vi "Climb (Piston) Controller.vi"(8 "error in":errorcluster) -> ()   [LabVIEW 2020]
doc: "This VI executes continuously carrying out the current operation and responding to updates or new operations. It will often contain the timing or control code that is difficult to place directly in TeleOp. This VI generally opens all sensors and motors and isolates the rest of the robot code from knowing how the operations are carried out."
uses:
  <vilib>/Rock Robotics/WPI/Framework/Completion Status.ctl
  Climb (Piston) Setpoints.ctl
  Climb (Piston) Operations.ctl
  <vilib>/Rock Robotics/WPI/Solenoid/WPI_SolenoidChannel.ctl
  <vilib>/Rock Robotics/WPI/Solenoid/WPI_SolenoidValue.ctl
  <vilib>/Rock Robotics/WPI/Solenoid/WPI_SolenoidOpenSingle.vi
  <vilib>/Rock Robotics/WPI/Solenoid/WPI_SolenoidSetEnum.vi
  <vilib>/Rock Robotics/Network Tables/NT Write Boolean.vi
panel:
  in  "Interactive Values":T1
  out "Current\nCmd":string
  in  "Buttons":cluster{"Execute Cmd":bool, "Abort Cmd":bool}
  out "Command Timing":cluster{"Start Time (ms)":u32, "Iterations":i32}
  out "Status":T3
  # "Tip: It may be helpful to observe inputs and sensor values.\nYou may also want to display tuning or debugging controls."
  # "Interactive Command: You may fill in the settings for a command\nand schedule it with the Execute button. You can observe and abort\nany command while fine tuning the code for the controller."
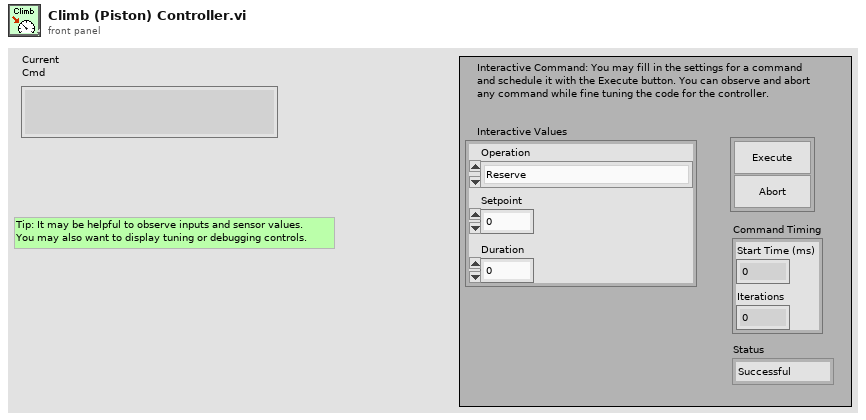
[diagram p1: front panel]
types:
  T1 = typedef "Climb (Piston) Setpoints.ctl" = cluster{"Operation":T2, "Setpoint":dbl, "Duration":dbl}
  T2 = typedef "Climb (Piston) Operations.ctl" = enum16{"Reserve", "Read Current", "Immediate", "Piston Up", "Piston Down"}
  T3 = typedef "Completion Status.ctl" = enum16{"Successful", "Aborted", "Incomplete"}
  T4 = typedef "WPI_SolenoidChannel.ctl" = enum8{"Solenoid 0", "Solenoid 1", "Solenoid 2", "Solenoid 3", "Solenoid 4", "Solenoid 5", "Solenoid 6", "Solenoid 7", "Solenoid 8", "Solenoid 9", "Solenoid 10", "Solenoid 11", "Solenoid 12", "Solenoid 13", "Solenoid 14", "Solenoid 15", "Invalid"}
  T5 = typedef "WPI_CompressorDevRef.ctl" = cluster{"DevStatus":errorcluster, "Pneumatics Control Module":u8}
  T6 = typedef "WPI_SolenoidDevRef.ctl" = cluster{"DevStatus":errorcluster, "Pneumatics Control Module":u8, "Forward Solenoid Channel":T4, "Reverse Solenoid Channel":T4}
  T7 = typedef "Command Status Info.ctl" = cluster{"Name":string, "Status":T3, "notifier out":T8}
  T8 = typedef "Completion Notifier.ctl" = refnum<notifier>
  T9 = cluster{"Current Command":T1, "Command Timing":cluster{"Start Time (ms)":u32, "Iterations":i32}, "Command Arguments":cluster{"Command Info":T7, "Description":string, "Default Command":T1, "queue out":refnum<queue>, "Subsystem Name":string}}
  T10 = typedef "WPI_SolenoidValue.ctl" = enum16{"Off", "On", "Forward", "Reverse"}
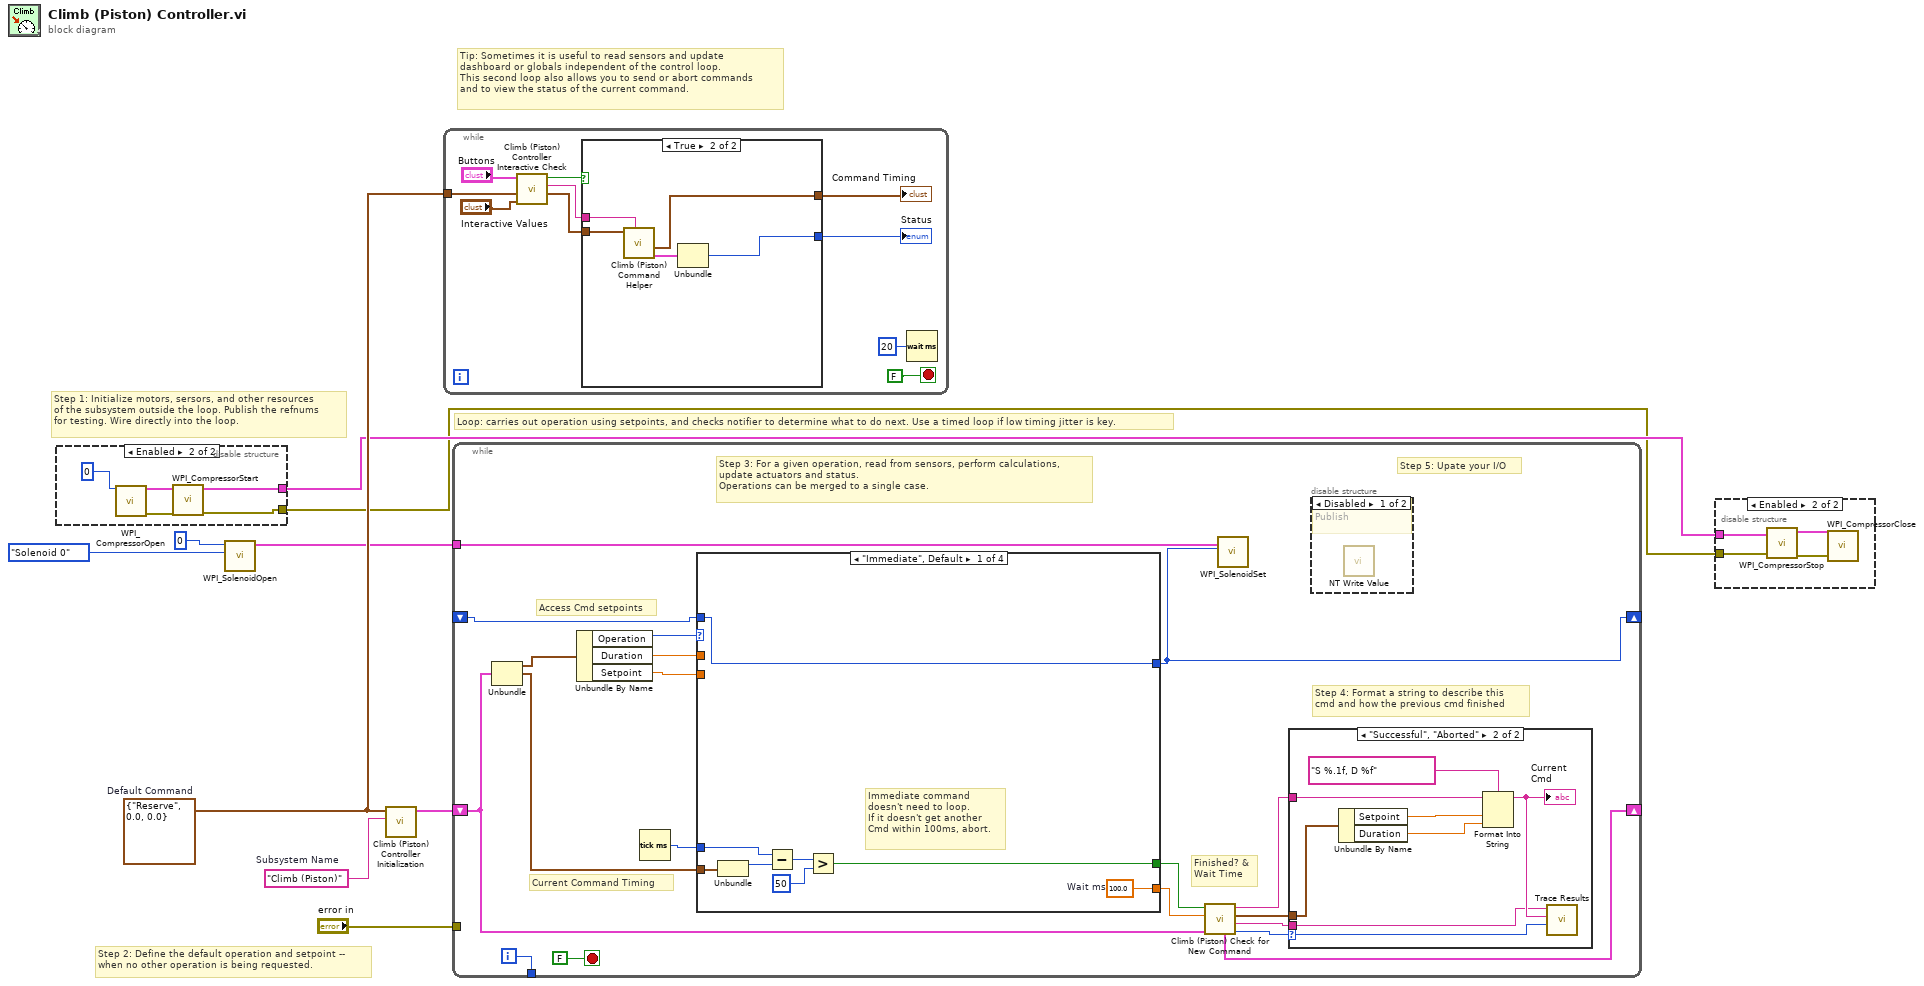
[diagram p0: block diagram]
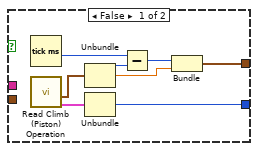
[diagram p4: hidden frame]
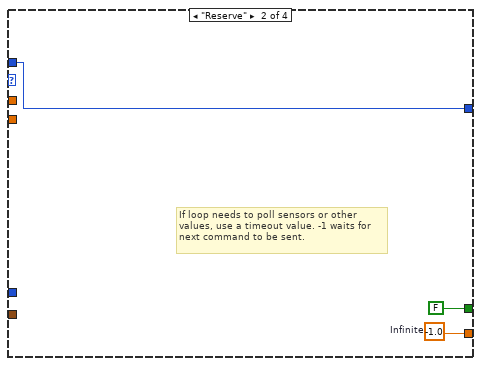
[diagram p7: hidden frame]
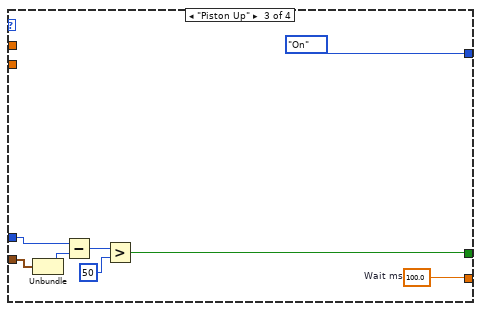
[diagram p8: hidden frame]
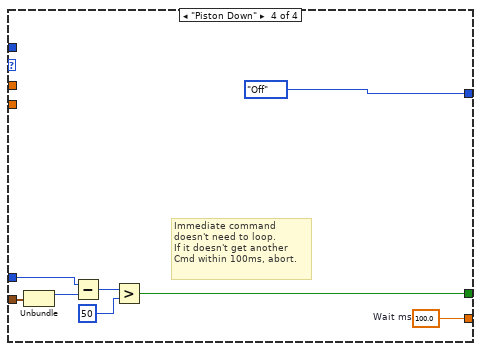
[diagram p9: hidden frame]
diagram:
  w6 = T1 {"Operation"=enum."Reserve", "Setpoint"=0.0, "Duration"=0.0}  # Default Command
  w7 = "Climb (Piston)"  # Subsystem Name
  # "Tip: Sometimes it is useful to read sensors and update\ndashboard or globals independent of the control loop.\nThis second loop also allows you to send or abort commands\nand to view the status of the current command."
  # "Step 2: Define the default operation and setpoint --\nwhen no other operation is being requested."
  # "Step 1: Initialize motors, sersors, and other resources\nof the subsystem outside the loop. Publish the refnums\nfor testing. Wire directly into the loop."
  # "Loop: carries out operation using setpoints, and checks notifier to determine what to do next. Use a timed loop if low timing jitter is key."
  n1 = disable-structure shown="Enabled" {
    disable-tunnel: [_ w12] -> w2
    disable-tunnel: [_ w11] -> w1
    frame Disabled {
    }
    frame Enabled {
      n2 = call <vilib>:"WPI_CompressorOpen.vi"("Pneumatics device (def)"=u8 0) -> ("CompressorDevRef"=w14:T5, "error out"=w13:errorcluster)  [unwired: 13 in]
      n3 = call <vilib>:"WPI_CompressorStart.vi"("error in (no error)"=w13, "CompressorDevRef"=w14) -> ("error out"=w11:errorcluster, "CompressorDevRef"=w12:T5)  [unwired: 8 in]
    }
  }
  n4 = call-poly <vilib>:"WPI_SolenoidOpen.vi"("Solenoid Channel"=WPI_SolenoidChannel."Solenoid 0", "Pneumatics Device (def)"=u8 0 ("Pneumatics Control Module (0)")) -> ("SolenoidDevRef"=w3:T6)  [unwired: 8 in, 1 out]
  n5 = call "Climb (Piston) Controller Initialization.vi"("Subsystem Name"=w7, "Default Command"=w6) -> ("Current Command"=w8:T9)  [unwired: 9 in]
  n6 = while {
    tunnel: w6 -> [w21]
    stop <- FALSE stop-if-true
    n7 = call "Climb (Piston) Controller Interactive Check.vi"("Interactive Command in"="Interactive Values", "Default Command"=w21, "Buttons"="Buttons") -> ("Interactive Command out"=w18:T1, "Trace String"=w19:string, "Schedule"=w20:bool)  [unwired: 6 in]
    n8 = case shown="True" w20 {
      tunnel: [w32 w37] -> w17
      tunnel: w18 -> [_ w35]
      tunnel: [w28 w33] -> w16
      tunnel: w19 -> [_ w36]
      frame False {
        n9 = Tick Count (ms)() -> (millisecond timer value=w27:u32)
        n10 = call "Read Climb (Piston) Operation.vi"() -> ("Command Info"=w25:T7, "SubSystem Data"=w26:T1)  [unwired: 9 in, 1 out]
        n11 = Unbundle(w26) -> ("Operation"=w31:T2, "Setpoint"=w29:dbl)  [unwired: 1 out]
        n12 = Unbundle(w25) -> ("Status"=w32:T3)  [unwired: 2 out]
        n13 = Subtract(x=w27, y=w31) -> (x-y=w30:u32)
        n14 = Bundle(w30, "Setpoint"=w29) -> (w28:cluster{u32, "Setpoint":dbl})  [unwired: 1 in]
      }
      frame True {
        n15 = call "Climb (Piston) Command Helper.vi"("Description"=w36, "SubSystem Data"=w35) -> ("Command Info Out"=w34:T7, "Command Timing"=w33:cluster{"Start Time (ms)":u32, "Iterations":i32})  [unwired: 7 in, 1 out]
        n16 = Unbundle(w34) -> ("Status"=w37:T3)  [unwired: 2 out]
      }
    }
    "Status" <- w17
    "Command Timing" <- w16
    n17 = Wait (ms)(milliseconds to wait=u32 20) -> ()  [unwired: 1 out]
  }
  n18 = while {
    shift-right: [w48] -> _
    shift-left: w8 -> [w41]
    tunnel: [w55] -> _
    tunnel: "error in" -> [_]
    tunnel: w3 -> [w40]
    shift-right: [w39] -> _
    shift-left: _ -> [w38]
    i -> [w55]
    stop <- FALSE stop-if-true
    # "Step 5: Upate your I/O"
    # "Step 4: Format a string to describe this\ncmd and how the previous cmd finished"
    # "Current Command Timing"
    # "Access Cmd setpoints"
    # "Finished? &\nWait Time"
    # "Step 3: For a given operation, read from sensors, perform calculations,\nupdate actuators and status.\nOperations can be merged to a single case."
    n19 = Unbundle(w41) -> ("Current Command"=w54:T1, "Command Timing"=w50:cluster{"Start Time (ms)":u32, "Iterations":i32})  [unwired: 1 out]
    n20 = Unbundle By Name(w54) -> ("Operation"=w53:T2, "Duration"=w52:dbl, "Setpoint"=w49:dbl)
    n21 = Tick Count (ms)() -> (millisecond timer value=w51:u32)
    n22 = case shown="\"Immediate\", Default" w53 {
      tunnel: [w72 w75 w77 w85] -> w46
      tunnel: [w66 FALSE ("ignore previous (F)") w78 w86] -> w47
      tunnel: w50 -> [w68 _ w81 w87]
      tunnel: w52 -> [_ _ _ _]
      tunnel: w51 -> [w67 _ w79 w89]
      tunnel: w49 -> [_ _ _ _]
      tunnel: [w65 w73 WPI_SolenoidValue."On" ("Value") WPI_SolenoidValue."Off" ("Value")] -> w39
      tunnel: w38 -> [w65 w73 _ _]
      frame "Immediate", Default {
        w72 = 100.0  # Wait ms
        # "Immediate command\ndoesn't need to loop.\nIf it doesn't get another\nCmd within 100ms, abort."
        n23 = Unbundle(w68) -> ("Start Time (ms)"=w71:u32)  [unwired: 1 out]
        n24 = Subtract(x=w67, y=w71) -> (x-y=w70:u32)
        n25 = Greater?(x=w70, y=u8 50 ("Left Motor")) -> (0:w66:bool)
      }
      frame "Reserve" {
        w75 = -1.0  # Infinite
        # "If loop needs to poll sensors or other\nvalues, use a timeout value. -1 waits for\nnext command to be sent."
      }
      frame "Piston Up" {
        w77 = 100.0  # Wait ms
        n26 = Unbundle(w81) -> ("Start Time (ms)"=w80:u32)  [unwired: 1 out]
        n27 = Subtract(x=w79, y=w80) -> (x-y=w83:u32)
        n28 = Greater?(x=w83, y=u8 50 ("Left Motor")) -> (0:w78:bool)
      }
      frame "Piston Down" {
        w85 = 100.0  # Wait ms
        # "Immediate command\ndoesn't need to loop.\nIf it doesn't get another\nCmd within 100ms, abort."
        n29 = Unbundle(w87) -> ("Start Time (ms)"=w88:u32)  [unwired: 1 out]
        n30 = Subtract(x=w89, y=w88) -> (x-y=w91:u32)
        n31 = Greater?(x=w91, y=u8 50 ("Left Motor")) -> (0:w86:bool)
      }
    }
    n32 = call "Climb (Piston) Check for New Command.vi"("Current Command"=w41, "Wait time (ms)"=w46, "Finished?"=w47) -> ("Completion"=w42:T3, "Subsystem Name"=w43:string, "Current Command"=w44:T1, "Initial Trace String"=w45:string, "NextCommand"=w48:T9)  [unwired: 4 in]
    n33 = call-poly <vilib>:"WPI_SolenoidSet.vi"("Value"=w39, "SolenoidDevRef"=w40) -> ()  [unwired: 8 in, 2 out]
    n34 = case shown="\"Successful\", \"Aborted\"" w42 {
      selector: w42 -> [_ w64]
      tunnel: w45 -> [_ w60]
      tunnel: w44 -> [_ w61]
      tunnel: w43 -> [_ w57]
      frame "Incomplete", Default {
        # "Continuing current command"
      }
      frame "Successful", "Aborted" {
        # "Report and setup for next command"
        n35 = Unbundle By Name(w61) -> ("Setpoint"=w63:dbl, "Duration"=w58:dbl)
        n36 = Format Into String(format string="S %.1f, D %f", initial string=w60, w63, w58) -> (resulting string=w59:string)  [unwired: 1 in, 1 out]
        "Current\nCmd" <- w59
        n37 = call <vilib>:"Trace Results.vi"("Status of previous command"=w64, "Description"=w59, "Subsystem"=w57) -> ()  [unwired: 9 in]
      }
    }
    n38 = disable-structure shown="Disabled" {
      frame Disabled {
        # "Publish"
        n39 = call-poly <vilib>:"NT Write Value.vi"() -> ()  [unwired: 11 in, 1 out]
      }
      frame Enabled {
      }
    }
  }
  n40 = disable-structure shown="Enabled" {
    disable-tunnel: w2 -> [_ w95]
    disable-tunnel: w1 -> [_ w93]
    frame Disabled {
    }
    frame Enabled {
      n41 = call <vilib>:"WPI_CompressorStop.vi"("error in (no error)"=w93, "CompressorDevRef"=w95) -> ("error out"=w92:errorcluster, "CompressorDevRef"=w94:T5)  [unwired: 8 in]
      n42 = call <vilib>:"WPI_CompressorClose.vi"("error in (no error)"=w92, "CompressorDevRef"=w94) -> ()  [unwired: 9 in, 1 out]
    }
  }
